vi "openMotor-83811664.vi"() -> (0 "Device":refnum<k24>, 1 ".NET Refnum out":refnum<k24>)   [LabVIEW 2014]
doc: "André Romero\nandretec@ifsc.usp.br"
uses:
  C:/UsersLab/AndreTec/LabView2014-32bits/kinesisTec/Kinesis/Thorlabs.MotionControl.Controls.dll
  Kinesis/Thorlabs.MotionControl.Controls.dll
  C:/UsersLab/AndreTec/LabView2014-32bits/kinesisTec/Kinesis/Thorlabs.MotionControl.TCube.DCServoCLI.dll
  Kinesis/Thorlabs.MotionControl.TCube.DCServoCLI.dll
panel:
  in  ".NET Refnum in":refnum<k24>(container)
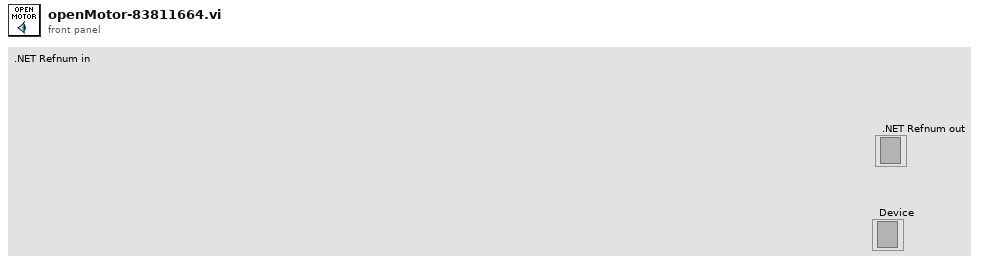
[diagram p1: front panel]
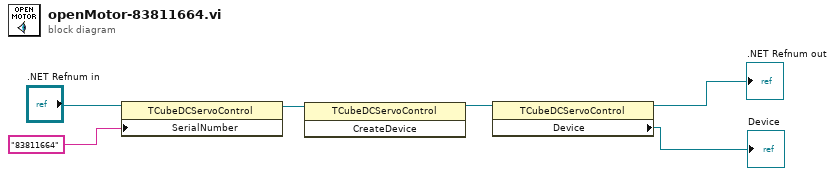
[diagram p0: block diagram]
diagram:
  n1 = property class="TCubeDCServoControl"(reference=".NET Refnum in", "SerialNumber"="83811664") -> (reference out=w4:refnum<k24>)  [unwired: 1 in, 1 out]
  n2 = invoke class="TCubeDCServoControl" method="CreateDevice"(reference=w4) -> (reference out=w5:refnum<k24>)  [unwired: 2 in, 2 out]
  n3 = property class="TCubeDCServoControl"(reference=w5) -> (reference out=→".NET Refnum out":refnum<k24>, "Device"=→"Device":refnum<k24>)  [unwired: 1 in, 1 out]
